vi "Particle Detection.vi"() -> ()   [LabVIEW 2014]
uses:
  <vilib>/vision/driver/NI_Vision_Acquisition_Software.lvlib
  <vilib>/userdefined/High Color/IMAQdx.ctl
panel:
  out "x-y":u32
  out "Before erosion":T1(plugin-control)
  out "Number of Particles after":i32
  out "After erosions":T1(plugin-control)
  in  "milliseconds to wait":u32
  out "Original":T1(plugin-control)
  in  "Number of Erosion":i32=2
  out "Number of Particles before":i32
  in  "stop":bool
  out "error out":errorcluster
  in  "error in (no error)":errorcluster
  in  "Image Name":string="webcam"
  in  "Session In":T2="cam0"
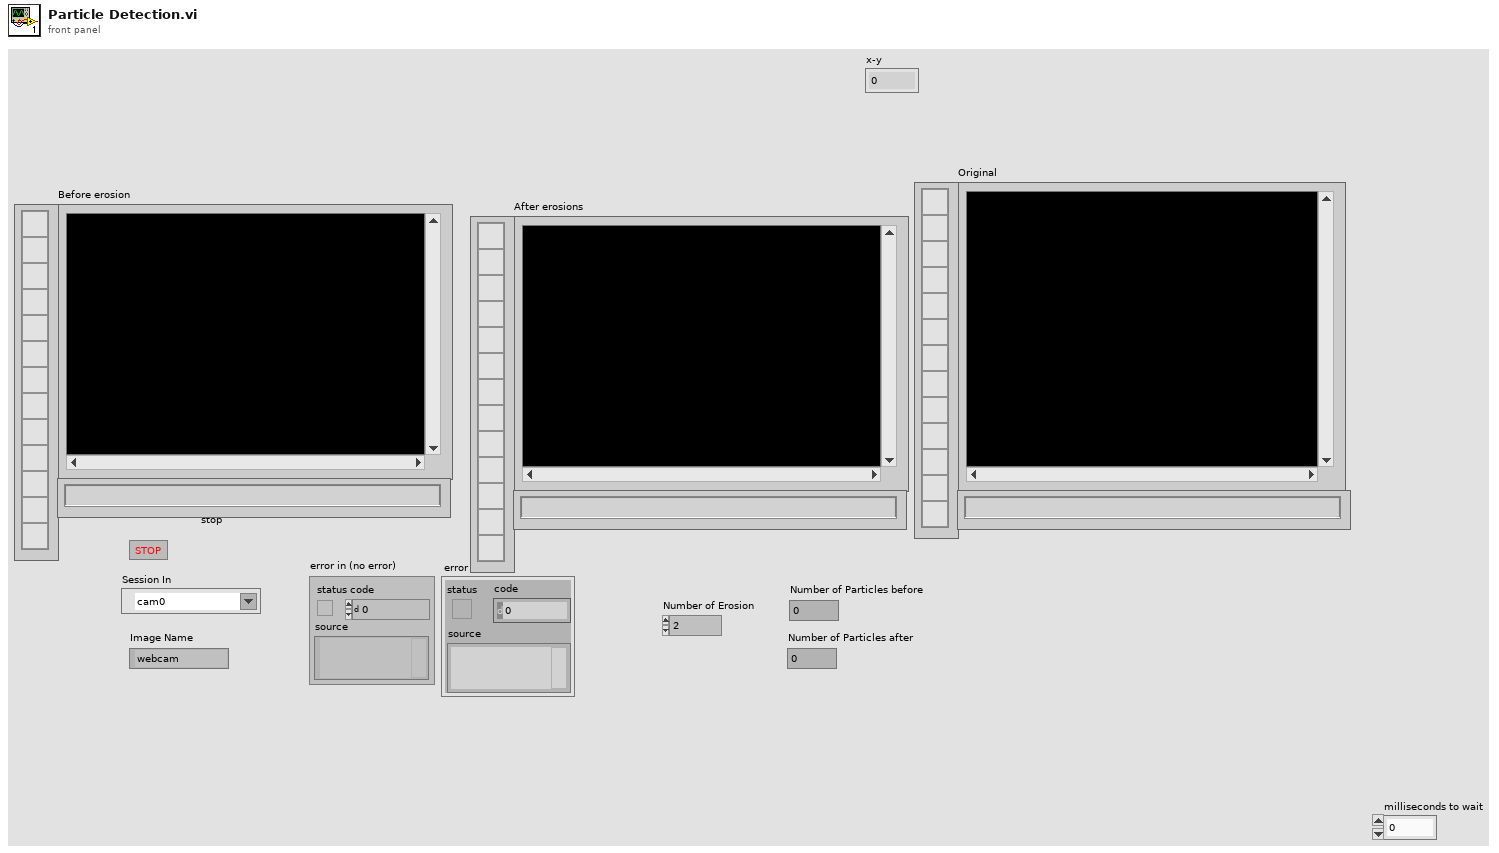
[diagram p1: front panel]
types:
  T1 = typedef "IMAQ Image.ctl" = refnum<image>
  T2 = typedef "IMAQdx.ctl" = refnum<k21>
  T3 = typedef "Image Type" = u32
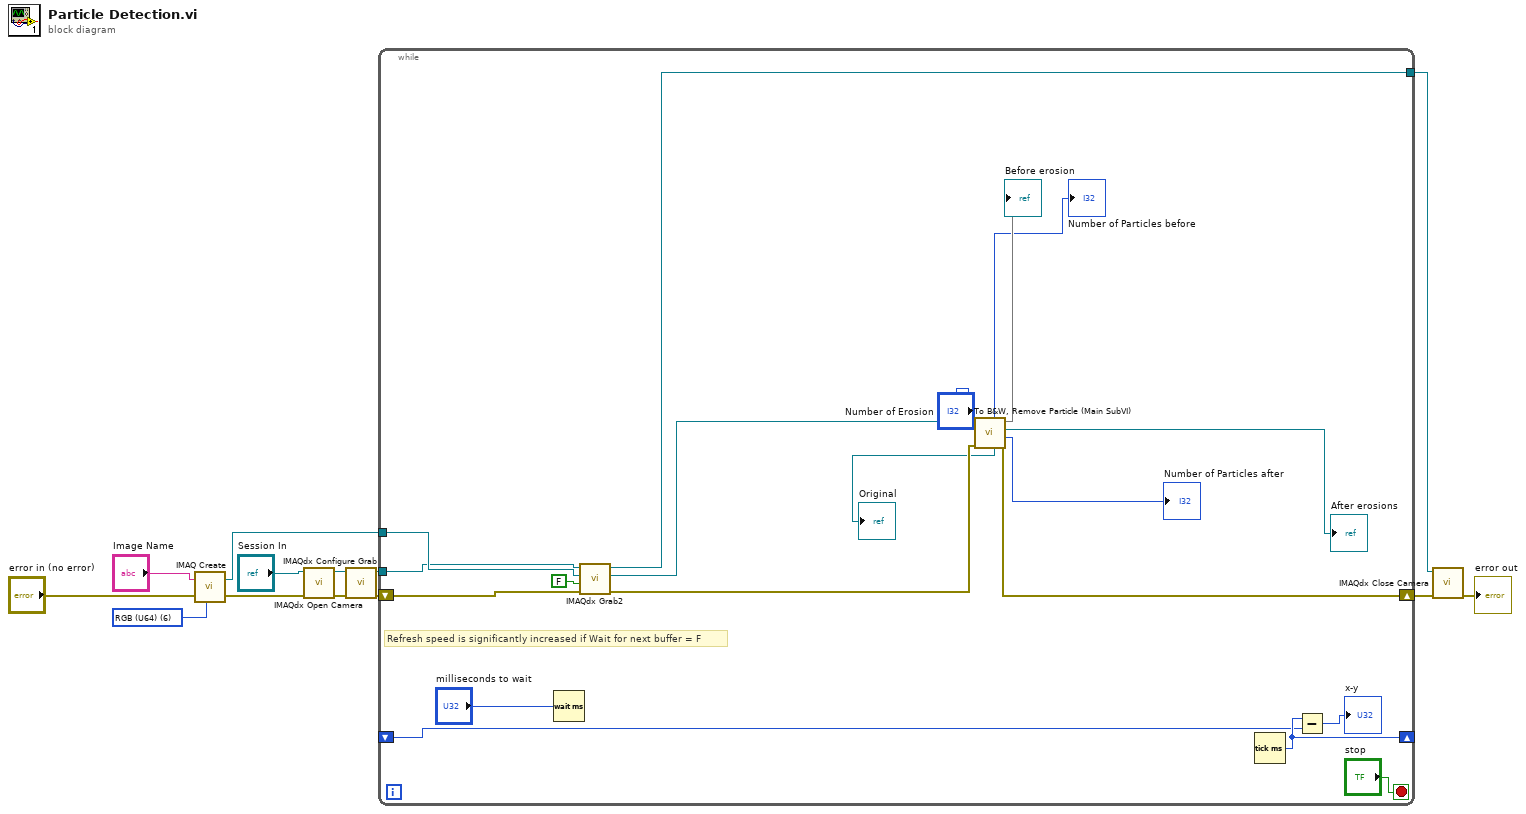
[diagram p0: block diagram]
diagram:
  w10 = T3 6 items=["Grayscale (U8)", "Grayscale (I16)", "Grayscale (SGL)", "Complex (CSG)", "RGB (U32)", "HSL (U32)", "RGB (U64)", "Grayscale (U16)"] ("Image Type")
  n1 = call "IMAQ Create"("Image Name"="Image Name", "Image Type"=w10, "error in (no error)"="error in (no error)") -> ("New Image"=w9:T1, "error out"=w7:errorcluster)  [unwired: 2 in]
  n2 = call <vilib>:"IMAQdx Open Camera.vi"("error in"=w7, "Session In"="Session In") -> ("error out"=w2:errorcluster, "Session Out"=w4:T2)  [unwired: 8 in]
  n3 = call <vilib>:"IMAQdx Configure Grab.vi"("error in"=w2, "Session In"=w4) -> ("error out"=w1:errorcluster, "Session Out"=w3:T2)  [unwired: 8 in]
  n4 = while {
    tunnel: w9 -> [w32]
    shift-right: [w22] -> w13
    shift-left: w1 -> [w29]
    tunnel: w3 -> [w30]
    tunnel: [w28] -> w11
    shift-right: [w21] -> _
    shift-left: _ -> [w20]
    stop <- "stop" stop-if-true
    # "Refresh speed is significantly increased if Wait for next buffer = F"
    n5 = Wait (ms)(milliseconds to wait="milliseconds to wait") -> ()  [unwired: 1 out]
    n6 = call <vilib>:"IMAQdx Grab2.vi"("error in"=w29, "Wait for Next Buffer? (Yes)"=FALSE, "Image In"=w32, "Session In"=w30) -> ("error out"=w27:errorcluster, "Image Out"=w25:T1, "Session Out"=w28:T2)  [unwired: 4 in, 1 out]
    n7 = call "To B&W, Remove Particle (Main SubVI).vi"("error in (no error)"=w27, "Number of Erosion"="Number of Erosion", "Refnum in"=w25) -> ("error out"=w22:errorcluster, "Number of Particles after"=→"Number of Particles after":i32, "Image Out"=→"After erosions":T1, 3:→"Before erosion", "Original"=→"Original":T1, "Number of Particles before"=→"Number of Particles before":i32)  [unwired: 2 in, 1 out]
    n8 = Tick Count (ms)() -> (millisecond timer value=w21:u32)
    n9 = Subtract(x=w21, y=w20) -> (x-y=→"x-y":u32)
  }
  n10 = call <vilib>:"IMAQdx Close Camera.vi"("error in"=w13, "Session In"=w11) -> ("error out"=→"error out":errorcluster)  [unwired: 9 in]
